vi "decode serial.vi"(11 "unsigned byte array":u8[](array[numeric])=[255, 233, 144, 5, 233, 0, 24, 89]) -> (2 "1":u32, 3 "0":u32)   [LabVIEW 2017]
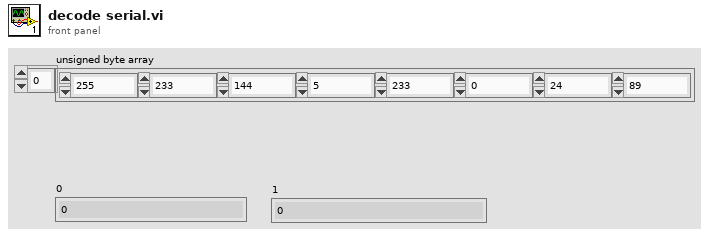
[diagram p1: front panel]
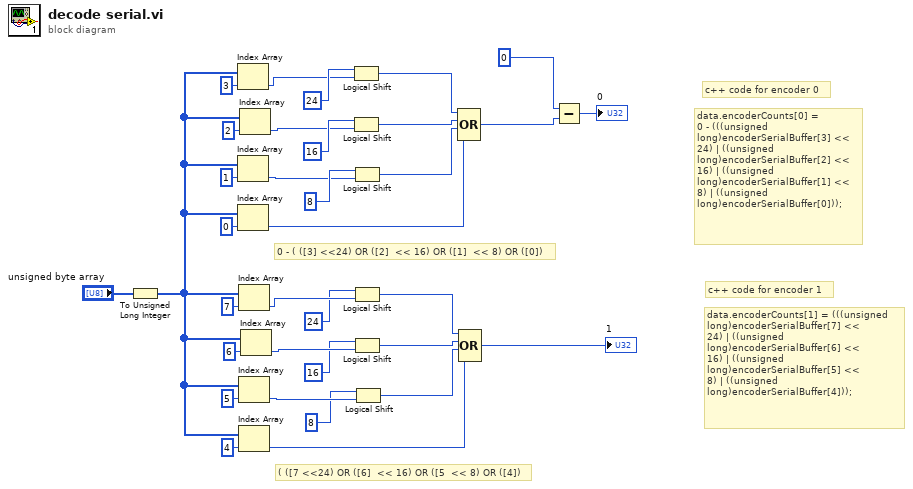
[diagram p0: block diagram]
diagram:
  # "( ([7 <<24) OR ([6]  << 16) OR ([5  << 8) OR ([4])"
  # "0 - ( ([3] <<24) OR ([2]  << 16) OR ([1]  << 8) OR ([0])"
  # "data.encoderCounts[1] = (((unsigned\nlong)encoderSerialBuffer[7] <<\n24) | ((unsigned\nlong)encoderSerialBuffer[6] <<\n16) | ((unsigned\nlong)encoderSerialBuffer[5] <<\n8) | ((unsigned\nlong)encoderSerialBuffer[4]));"
  # "c++ code for encoder 1"
  # "c++ code for encoder 0"
  # "data.encoderCounts[0] =\n0 - (((unsigned\nlong)encoderSerialBuffer[3] <<\n24) | ((unsigned\nlong)encoderSerialBuffer[2] <<\n16) | ((unsigned\nlong)encoderSerialBuffer[1] <<\n8) | ((unsigned\nlong)encoderSerialBuffer[0]));"
  n1 = To Unsigned Long Integer(number="unsigned byte array") -> (unsigned 32bit integer=w2:u32[])
  n2 = Index Array(array=w2, index=3) -> (element=w29:u32)
  n3 = Index Array(array=w2, index=1) -> (element=w24:u32)
  n4 = Index Array(array=w2, index=0) -> (element=w20:u32)
  n5 = Index Array(array=w2, index=7) -> (element=w7:u32)
  n6 = Index Array(array=w2, index=5) -> (element=w12:u32)
  n7 = Index Array(array=w2, index=4) -> (element=w16:u32)
  n8 = Index Array(array=w2, index=2) -> (element=w25:u32)
  n9 = Index Array(array=w2, index=6) -> (element=w11:u32)
  n10 = Logical Shift(y=24, x=w29) -> (x << y=w23:u32)
  n11 = Logical Shift(y=16, x=w25) -> (x << y=w22:u32)
  n12 = Logical Shift(y=8, x=w24) -> (x << y=w21:u32)
  n13 = Logical Shift(y=24, x=w7) -> (x << y=w13:u32)
  n14 = Logical Shift(y=16, x=w11) -> (x << y=w14:u32)
  n15 = Logical Shift(y=8, x=w12) -> (x << y=w15:u32)
  n16 = Compound Arithmetic op=OR(w23, w22, w21, w20) -> (w18:u32)
  n17 = Compound Arithmetic op=OR(w13, w14, w15, w16) -> (→"1":u32)
  n18 = Subtract(x=u32 0, y=w18) -> (x-y=→"0":u32)
